vi "WritePortStatus.vi"(8 "error in (no error)":errorcluster, 9 "Value":string, 10 "Port":dbl, 11 "Simulado in":refnum<class "Simulado.lvclass">) -> (0 "error out":errorcluster, 3 "Simulado out":refnum<class "Simulado.lvclass">)   [LabVIEW 2020, in "Simulado.lvclass"]
uses:
  Simulado.lvclass
  Simulado.lvclass/Simulado.ctl
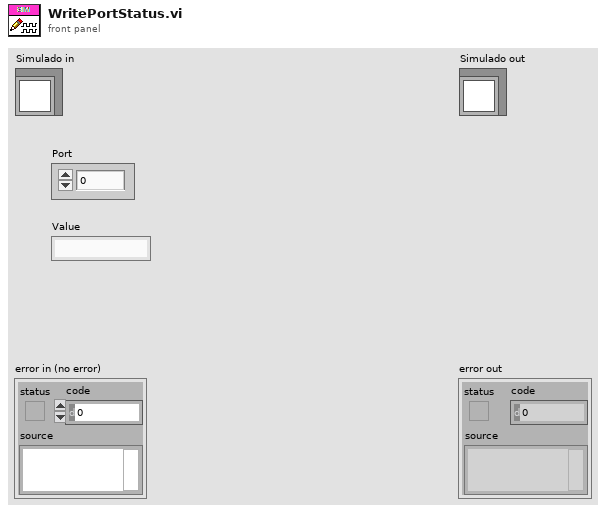
[diagram p1: front panel]
types:
  T1 = enum16{"Get Parameters", "Set Parameters", "Reset"}
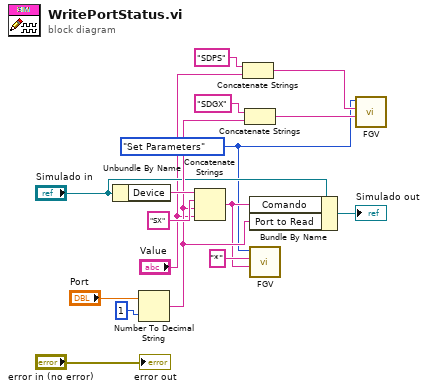
[diagram p0: block diagram]
diagram:
  w1 = T1."Set Parameters" ("Función")
  n1 = Unbundle By Name("Simulado in") -> ("Device"=w14:string)
  n2 = Number To Decimal String(number="Port", width (-)=i16 1) -> (decimal integer string=w11:string)
  n3 = Concatenate Strings(w14, "SX" ("string"), w11, "Value") -> (w4:string)
  n4 = Concatenate Strings("SDPS" ("string"), "Value") -> (w2:string)
  n5 = Concatenate Strings("SDGX" ("string"), w11) -> (w3:string)
  n6 = Bundle By Name(cluster="Simulado in", "Comando"=w4, "Port to Read"=w11) -> (→"Simulado out":refnum<class "Simulado.lvclass">)
  n7 = call "FGV.vi"("Comandos"=w4, "Respuestas"="*", "Función"=w1) -> ()  [unwired: 8 in, 1 out]
  n8 = call "FGV.vi"("Comandos"=w3, "Respuestas"=w2, "Función"=w1) -> ()  [unwired: 8 in, 1 out]
  "error out" <- "error in (no error)"
